vi "example.vi"   [LabVIEW 2019]
uses:
  write_command_reset.vi
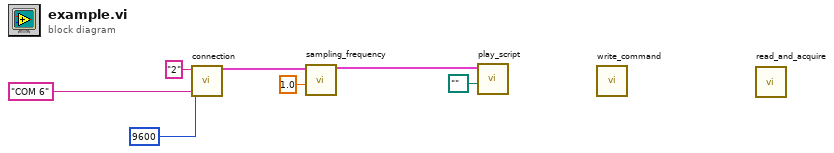
[diagram p0: block diagram]
diagram:
  n1 = call "connection.vi"("BAUD"=9600, "COM PORT"="COM 6", "GPIB address"="2") -> ("Connection"=w4:cluster{"queue out":refnum<queue>})  [unwired: 8 in]
  n2 = call "sampling_frequency.vi"("SF [Hz]"=1.0, "Connection"=w4) -> ("Connection 2"=w2:cluster{"queue out":refnum<queue>})  [unwired: 9 in]
  n3 = call "play_script.vi"("Path Script"=path "", "Connection"=w2) -> ()  [unwired: 9 in, 1 out]
  n4 = call-poly "write_command.vi"() -> ()  [unwired: 12 in]
  n5 = call "read_and_acquire.vi"() -> ()  [unwired: 12 in]
